vi "ClusterwitharrayBoolean.vi"(1 "Cluster In":cluster{"Array In":bool[], "Boolean In":bool}) -> (0 "Cluster Out":cluster{"Array Out":bool[], "Boolean out":bool})   [LabVIEW 2010]
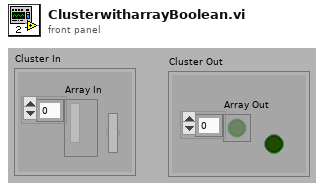
[diagram p1: front panel]
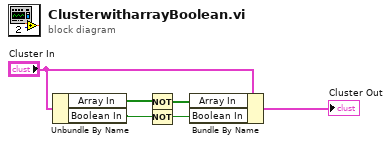
[diagram p0: block diagram]
diagram:
  n1 = Unbundle By Name("Cluster In") -> ("Array In"=w2:bool[], "Boolean In"=w3:bool)
  n2 = Not(x=w2) -> (.not. x?=w1:bool[])
  n3 = Not(x=w3) -> (.not. x?=w4:bool)
  n4 = Bundle By Name(cluster="Cluster In", "Array In"=w1, "Boolean In"=w4) -> (→"Cluster Out":cluster{"Array In":bool[], "Boolean In":bool})
